vi "App - analyze RUS V6.vi"() -> ()   [LabVIEW 2018] (continued)
"4corners"={"z (-pi/2)"=0.15435451062845643-0.4678200604991372i, "z(inf)"=0.4758200604991372+0.1223545106284564i, "z (pi/2)"=-0.11435451062845639+0.4438200604991372i, "z center"=0.020000000000000018-0.01200000000000001i, "z(0)"=-0.4358200604991372-0.14635451062845642i, "radius"=0.47520844066540857}}, "timestamp(min)"=87.08333333581686, "timestamp"=timestamp(3493733046 s since 1904-01-01), "Magn Field(T)"=0.0}, {"temperature"=210.861, "lorentzian"={"A (VHz)"=0.00034396524768400054, "f (Hz)"=664.2981443004336, "G (Hz)"=0.1690212753358618, "phi(rad)"=-1.2881319002414702, "Q"=3930.2634711541978, "Norm  Ampl"=0.08263262968234714, "bg (V)"=0.48948770996611757+0.12435861413405644i, "4corners"={"z (-pi/2)"=0.15635861413405647-0.48148770996611756i, "z(inf)"=0.48948770996611757+0.12435861413405644i, "z (pi/2)"=-0.11635861413405643+0.45748770996611754i, "z center"=0.020000000000000018-0.01200000000000001i, "z(0)"=-0.44948770996611753-0.14835861413405646i, "radius"=0.488888925480819}}, "timestamp(min)"=88.41666666418314, "timestamp"=timestamp(3493733126 s since 1904-01-01), "Magn Field(T)"=0.0}, {"temperature"=210.594, "lorentzian"={"A (VHz)"=0.0003323733612583622, "f (Hz)"=664.3188476258067, "G (Hz)"=0.16344657299552573, "phi(rad)"=-1.2279818487580703, "Q"=4064.4403577919747, "Norm  Ampl"=0.0788865424699876, "bg (V)"=0.48256027530198187+0.1582356056642887i, "4corners"={"z (-pi/2)"=0.19023560566428874-0.45856027530198185i, "z(inf)"=0.48256027530198187+0.1582356056642887i, "z (pi/2)"=-0.1342356056642887+0.45056027530198184i, "z center"=0.028000000000000025-0.0040000000000000036i, "z(0)"=-0.4265602753019818-0.16623560566428872i, "radius"=0.4826442122597888}}, "timestamp(min)"=89.73333333432674, "timestamp"=timestamp(3493733205 s since 1904-01-01), "Magn Field(T)"=0.0}, {"temperature"=210.336, "lorentzian"={"A (VHz)"=0.00033438773859277484, "f (Hz)"=664.3335964907527, "G (Hz)"=0.16118690371722072, "phi(rad)"=-1.2664496122682602, "Q"=4121.510998537639, "Norm  Ampl"=0.07822762004975677, "bg (V)"=0.4990184327589342+0.13343656181766148i, "4corners"={"z (-pi/2)"=0.18143656181766152-0.4750184327589342i, "z(inf)"=0.4990184327589342+0.13343656181766148i, "z (pi/2)"=-0.10943656181766145+0.45101843275893416i, "z center"=0.03600000000000003-0.01200000000000001i, "z(0)"=-0.42701843275893414-0.1574365618176615i, "radius"=0.4853224315729514}}, "timestamp(min)"=91.0666666701436, "timestamp"=timestamp(3493733285 s since 1904-01-01), "Magn Field(T)"=0.0}, {"temperature"=210.064, "lorentzian"={"A (VHz)"=0.0003264846409159807, "f (Hz)"=664.3536063641833, "G (Hz)"=0.1553160001327941, "phi(rad)"=-1.220684561377293, "Q"=4277.431853744402, "Norm  Ampl"=0.07467473957671357, "bg (V)"=0.4956247544092579+0.16091310841247816i, "4corners"={"z (-pi/2)"=0.2089131084124782-0.45562475440925787i, "z(inf)"=0.4956247544092579+0.16091310841247816i, "z (pi/2)"=-0.12091310841247813+0.44762475440925786i, "z center"=0.04400000000000004-0.0040000000000000036i, "z(0)"=-0.40762475440925783-0.16891310841247817i, "radius"=0.48079231703666836}}, "timestamp(min)"=92.38333333283663, "timestamp"=timestamp(3493733364 s since 1904-01-01), "Magn Field(T)"=0.0}, {"temperature"=209.8, "lorentzian"={"A (VHz)"=0.00033137804714622845, "f (Hz)"=664.3711441248129, "G (Hz)"=0.15484911121026917, "phi(rad)"=-1.2383855845330038, "Q"=4290.442088638566, "Norm  Ampl"=0.07481204115039657, "bg (V)"=0.49268141450734+0.16165586720424824i, "4corners"={"z (-pi/2)"=0.19365586720424827-0.45268141450733995i, "z(inf)"=0.49268141450734+0.16165586720424824i, "z (pi/2)"=-0.1216558672042482+0.46068141450733996i, "z center"=0.03600000000000003+0.0040000000000000036i, "z(0)"=-0.4206814145073399-0.15365586720424823i, "radius"=0.4831286441729039}}, "timestamp(min)"=93.70000000298023, "timestamp"=timestamp(3493733443 s since 1904-01-01), "Magn Field(T)"=0.0}, {"temperature"=209.539, "lorentzian"={"A (VHz)"=0.00035137190295300166, "f (Hz)"=664.3886135894766, "G (Hz)"=0.1587677742828772, "phi(rad)"=-1.2908942860300243, "Q"=4184.656594138132, "Norm  Ampl"=0.07809203185267653, "bg (V)"=0.5007211548751844+0.1478828779205012i, "4corners"={"z (-pi/2)"=0.1638828779205012-0.4607211548751844i, "z(inf)"=0.5007211548751844+0.1478828779205012i, "z (pi/2)"=-0.10788287792050116+0.4847211548751844i, "z center"=0.028000000000000025+0.01200000000000001i, "z(0)"=-0.4447211548751844-0.12388287792050118i, "radius"=0.49186323991378533}}, "timestamp(min)"=95.03333333134651, "timestamp"=timestamp(3493733523 s since 1904-01-01), "Magn Field(T)"=0.0}, {"temperature"=209.267, "lorentzian"={"A (VHz)"=0.0003551473471126149, "f (Hz)"=664.4069577109009, "G (Hz)"=0.15724780606018676, "phi(rad)"=-1.2959877034042098, "Q"=4225.222433034127, "Norm  Ampl"=0.07756980531564582, "bg (V)"=0.5027866875931508+0.14586231534066638i, "4corners"={"z (-pi/2)"=0.1618623153406664-0.46278668759315084i, "z(inf)"=0.5027866875931508+0.14586231534066638i, "z (pi/2)"=-0.10586231534066634+0.48678668759315086i, "z center"=0.028000000000000025+0.01200000000000001i, "z(0)"=-0.4467866875931508-0.12186231534066636i, "radius"=0.4932965823762012}}, "timestamp(min)"=96.35000000149012, "timestamp"=timestamp(3493733602 s since 1904-01-01), "Magn Field(T)"=0.0}, {"temperature"=209.008, "lorentzian"={"A (VHz)"=0.00035824718774550096, "f (Hz)"=664.4245585272355, "G (Hz)"=0.1570614171905534, "phi(rad)"=-1.3013567474955483, "Q"=4230.348677684018, "Norm  Ampl"=0.0778321762150261, "bg (V)"=0.5056730676055248+0.14391175019997515i, "4corners"={"z (-pi/2)"=0.15991175019997517-0.4656730676055247i, "z(inf)"=0.5056730676055248+0.14391175019997515i, "z (pi/2)"=-0.10391175019997512+0.4896730676055247i, "z center"=0.028000000000000025+0.01200000000000001i, "z(0)"=-0.44967306760552467-0.11991175019997513i, "radius"=0.4955524890024192}}, "timestamp(min)"=97.68333333730698, "timestamp"=timestamp(3493733682 s since 1904-01-01), "Magn Field(T)"=0.0}, {"temperature"=208.737, "lorentzian"={"A (VHz)"=0.0003620389778047644, "f (Hz)"=664.4414683185125, "G (Hz)"=0.1572813330614881, "phi(rad)"=-1.315732030850954, "Q"=4224.5411797136385, "Norm  Ampl"=0.07555321252410724, "bg (V)"=0.49282849367948844+0.10120097940000432i, "4corners"={"z (-pi/2)"=0.14920097940000437-0.48482849367948844i, "z(inf)"=0.49282849367948844+0.10120097940000432i, "z (pi/2)"=-0.09320097940000431+0.4448284936794884i, "z center"=0.028000000000000025-0.020000000000000018i, "z(0)"=-0.4368284936794884-0.14120097940000437i, "radius"=0.48036986369240786}}, "timestamp(min)"=99.0, "timestamp"=timestamp(3493733761 s since 1904-01-01), "Magn Field(T)"=0.0}, {"temperature"=208.465, "lorentzian"={"A (VHz)"=0.00036334054298061894, "f (Hz)"=664.4601452577426, "G (Hz)"=0.1577653201754836, "phi(rad)"=-1.3227956670777963, "Q"=4211.699659460383, "Norm  Ampl"=0.07315531107366603, "bg (V)"=0.4775102835579108+0.08582198624427292i, "4corners"={"z (-pi/2)"=0.14182198624427297-0.4775102835579108i, "z(inf)"=0.4775102835579108+0.08582198624427292i, "z (pi/2)"=-0.08582198624427292+0.42151028355791076i, "z center"=0.028000000000000025-0.028000000000000025i, "z(0)"=-0.42151028355791076-0.14182198624427297i, "radius"=0.4636970342550239}}, "timestamp(min)"=100.3166666701436, "timestamp"=timestamp(3493733840 s since 1904-01-01), "Magn Field(T)"=0.0}, {"temperature"=208.205, "lorentzian"={"A (VHz)"=0.0003655921916337196, "f (Hz)"=664.4796852677678, "G (Hz)"=0.15525145365190737, "phi(rad)"=-1.2967215976941358, "Q"=4280.02230985619, "Norm  Ampl"=0.07716533206824039, "bg (V)"=0.5064832255059715+0.13852553307676524i, "4corners"={"z (-pi/2)"=0.16252553307676526-0.4744832255059715i, "z(inf)"=0.5064832255059715+0.13852553307676524i, "z (pi/2)"=-0.10652553307676521+0.4824832255059715i, "z center"=0.028000000000000025+0.0040000000000000036i, "z(0)"=-0.4504832255059715-0.13052553307676523i, "radius"=0.49703452208089755}}, "timestamp(min)"=101.64999999850988, "timestamp"=timestamp(3493733920 s since 1904-01-01), "Magn Field(T)"=0.0}, {"temperature"=207.933, "lorentzian"={"A (VHz)"=0.0003696196043564403, "f (Hz)"=664.4980076667935, "G (Hz)"=0.1551610073255388, "phi(rad)"=-1.3004917013710942, "Q"=4282.635303292595, "Norm  Ampl"=0.07717961611290688, "bg (V)"=0.5073549264995896+0.13682259753273826i, "4corners"={"z (-pi/2)"=0.16082259753273828-0.4753549264995896i, "z(inf)"=0.5073549264995896+0.13682259753273826i, "z (pi/2)"=-0.10482259753273823+0.4833549264995896i, "z center"=0.028000000000000025+0.0040000000000000036i, "z(0)"=-0.4513549264995896-0.12882259753273825i, "radius"=0.49741631253384794}}, "timestamp(min)"=102.96666666865349, "timestamp"=timestamp(3493733999 s since 1904-01-01), "Magn Field(T)"=0.0}, {"temperature"=207.67, "lorentzian"={"A (VHz)"=0.0003688314220528578, "f (Hz)"=664.5154310442224, "G (Hz)"=0.15247576110630867, "phi(rad)"=-1.3185668128316879, "Q"=4358.170939582397, "Norm  Ampl"=0.07594365786598505, "bg (V)"=0.5103106326617382+0.12830020642125523i, "4corners"={"z (-pi/2)"=0.15230020642125525-0.47831063266173807i, "z(inf)"=0.5103106326617382+0.12830020642125523i, "z (pi/2)"=-0.09630020642125518+0.4863106326617381i, "z center"=0.028000000000000025+0.0040000000000000036i, "z(0)"=-0.45431063266173805-0.1203002064212552i, "radius"=0.4980703642006144}}, "timestamp(min)"=104.28333333134651, "timestamp"=timestamp(3493734078 s since 1904-01-01), "Magn Field(T)"=0.0}, {"temperature"=207.397, "lorentzian"={"A (VHz)"=0.00037157271400023234, "f (Hz)"=664.5338643964093, "G (Hz)"=0.15192949142637535, "phi(rad)"=-1.3189009092108237, "Q"=4373.962277879675, "Norm  Ampl"=0.07614323738836301, "bg (V)"=0.5133586305123503+0.1289128189052309i, "4corners"={"z (-pi/2)"=0.15291281890523092-0.4813586305123502i, "z(inf)"=0.5133586305123503+0.1289128189052309i, "z (pi/2)"=-0.09691281890523087+0.48935863051235023i, "z center"=0.028000000000000025+0.0040000000000000036i, "z(0)"=-0.4573586305123502-0.1209128189052309i, "radius"=0.5011748323087215}}, "timestamp(min)"=105.61666666716337, "timestamp"=timestamp(3493734158 s since 1904-01-01), "Magn Field(T)"=0.0}, {"temperature"=207.121, "lorentzian"={"A (VHz)"=0.00037560722465557504, "f (Hz)"=664.5517885931691, "G (Hz)"=0.15163343901734644, "phi(rad)"=-1.3231000954626153, "Q"=4382.620303936695, "Norm  Ampl"=0.07591961547744219, "bg (V)"=0.5133977788844358+0.12675194644126214i, "4corners"={"z (-pi/2)"=0.15075194644126216-0.4813977788844358i, "z(inf)"=0.5133977788844358+0.12675194644126214i, "z (pi/2)"=-0.09475194644126211+0.4893977788844358i, "z center"=0.028000000000000025+0.0040000000000000036i, "z(0)"=-0.4573977788844358-0.11875194644126214i, "radius"=0.5006785836253256}}, "timestamp(min)"=106.93333333730698, "timestamp"=timestamp(3493734237 s since 1904-01-01), "Magn Field(T)"=0.0}, {"temperature"=206.86, "lorentzian"={"A (VHz)"=0.00037939817093463887, "f (Hz)"=664.5704803534437, "G (Hz)"=0.1507306425391779, "phi(rad)"=-1.3256025377721956, "Q"=4408.9938791358145, "Norm  Ampl"=0.07554516623773996, "bg (V)"=0.514202618763606+0.12566179261706728i, "4corners"={"z (-pi/2)"=0.1496617926170673-0.48220261876360593i, "z(inf)"=0.514202618763606+0.12566179261706728i, "z (pi/2)"=-0.09366179261706727+0.49020261876360594i, "z center"=0.028000000000000025+0.0040000000000000036i, "z(0)"=-0.4582026187636059-0.11766179261706729i, "radius"=0.5011931546573503}}, "timestamp(min)"=108.26666666567326, "timestamp"=timestamp(3493734317 s since 1904-01-01), "Magn Field(T)"=0.0}, {"temperature"=206.586, "lorentzian"={"A (VHz)"=0.0003799233187956319, "f (Hz)"=664.588180324614, "G (Hz)"=0.14905726588662013, "phi(rad)"=-1.3374419748250967, "Q"=4458.609758950835, "Norm  Ampl"=0.07486814015789056, "bg (V)"=0.5166640632352237+0.12014782699526805i, "4corners"={"z (-pi/2)"=0.14414782699526807-0.48466406323522376i, "z(inf)"=0.5166640632352237+0.12014782699526805i, "z (pi/2)"=-0.08814782699526802+0.49266406323522377i, "z center"=0.028000000000000025+0.0040000000000000036i, "z(0)"=-0.46066406323522374-0.11214782699526804i, "radius"=0.5022776965118813}}, "timestamp(min)"=109.58333333581686, "timestamp"=timestamp(3493734396 s since 1904-01-01), "Magn Field(T)"=0.0}, {"temperature"=206.322, "lorentzian"={"A (VHz)"=0.00038342258394746456, "f (Hz)"=664.6064246538435, "G (Hz)"=0.14844526330238045, "phi(rad)"=-1.342088405083977, "Q"=4477.114391316425, "Norm  Ampl"=0.0747010798065654, "bg (V)"=0.5181192065643716+0.11809037028339893i, "4corners"={"z (-pi/2)"=0.14209037028339894-0.4861192065643716i, "z(inf)"=0.5181192065643716+0.11809037028339893i, "z (pi/2)"=-0.0860903702833989+0.4941192065643716i, "z center"=0.028000000000000025+0.0040000000000000036i, "z(0)"=-0.46211920656437155-0.11009037028339892i, "radius"=0.5032230611117621}}, "timestamp(min)"=110.89999999850988, "timestamp"=timestamp(3493734475 s since 1904-01-01), "Magn Field(T)"=0.0}, {"temperature"=206.047, "lorentzian"={"A (VHz)"=0.00038522781206593883, "f (Hz)"=664.6239877084581, "G (Hz)"=0.1476327330726419, "phi(rad)"=-1.3521683622314384, "Q"=4501.874170286026, "Norm  Ampl"=0.0739234746791219, "bg (V)"=0.5168062088247101+0.11260258100289335i, "4corners"={"z (-pi/2)"=0.13660258100289335-0.48480620882471004i, "z(inf)"=0.5168062088247101+0.11260258100289335i, "z (pi/2)"=-0.08060258100289332+0.49280620882471005i, "z center"=0.028000000000000025+0.0040000000000000036i, "z(0)"=-0.46080620882471-0.10460258100289334i, "radius"=0.5007255040299785}}, "timestamp(min)"=112.23333333432674, "timestamp"=timestamp(3493734555 s since 1904-01-01), "Magn Field(T)"=0.0}, {"temperature"=205.772, "lorentzian"={"A (VHz)"=0.00038879314280680584, "f (Hz)"=664.6422601490035, "G (Hz)"=0.14766020358391277, "phi(rad)"=-1.3505384031514258, "Q"=4501.160394048208, "Norm  Ampl"=0.07402344475594164, "bg (V)"=0.5171983096693449+0.1135267359741549i, "4corners"={"z (-pi/2)"=0.13752673597415493-0.4851983096693449i, "z(inf)"=0.5171983096693449+0.1135267359741549i, "z (pi/2)"=-0.08152673597415487+0.4931983096693449i, "z center"=0.028000000000000025+0.0040000000000000036i, "z(0)"=-0.4611983096693449-0.10552673597415489i, "radius"=0.5013093776067794}}, "timestamp(min)"=113.55000000447035, "timestamp"=timestamp(3493734634 s since 1904-01-01), "Magn Field(T)"=0.0}, {"temperature"=205.505, "lorentzian"={"A (VHz)"=0.0003927838145535556, "f (Hz)"=664.6602601074228, "G (Hz)"=0.14759958362580006, "phi(rad)"=-1.3539126044269483, "Q"=4503.130996578515, "Norm  Ampl"=0.07397858406419787, "bg (V)"=0.5174693417428737+0.1118543640956627i, "4corners"={"z (-pi/2)"=0.1358543640956627-0.4854693417428737i, "z(inf)"=0.5174693417428737+0.1118543640956627i, "z (pi/2)"=-0.07985436409566267+0.4934693417428737i, "z center"=0.028000000000000025+0.0040000000000000036i, "z(0)"=-0.4614693417428737-0.10385436409566269i, "radius"=0.5012113330329651}}, "timestamp(min)"=114.86666666716337, "timestamp"=timestamp(3493734713 s since 1904-01-01), "Magn Field(T)"=0.0}, {"temperature"=205.23, "lorentzian"={"A (VHz)"=0.0003935754582975437, "f (Hz)"=664.6782562264044, "G (Hz)"=0.14661811059554475, "phi(rad)"=-1.3514260691358269, "Q"=4533.39804698453, "Norm  Ampl"=0.07351191973354369, "bg (V)"=0.5173678077971541+0.11310860545837348i, "4corners"={"z (-pi/2)"=0.1371086054583735-0.48536780779715405i, "z(inf)"=0.5173678077971541+0.11310860545837348i, "z (pi/2)"=-0.08110860545837345+0.49336780779715406i, "z center"=0.028000000000000025+0.0040000000000000036i, "z(0)"=-0.46136780779715403-0.10510860545837347i, "radius"=0.5013836246760193}}, "timestamp(min)"=116.20000000298023, "timestamp"=timestamp(3493734793 s since 1904-01-01), "Magn Field(T)"=0.0}, {"temperature"=204.949, "lorentzian"={"A (VHz)"=0.000399394876662407, "f (Hz)"=664.6963935252326, "G (Hz)"=0.1471833400427258, "phi(rad)"=-1.3610534018832139, "Q"=4516.111628750089, "Norm  Ampl"=0.07359368008705944, "bg (V)"=0.5170555937119127+0.10810707626710435i, "4corners"={"z (-pi/2)"=0.13210707626710438-0.48505559371191265i, "z(inf)"=0.5170555937119127+0.10810707626710435i, "z (pi/2)"=-0.07610707626710432+0.49305559371191265i, "z center"=0.028000000000000025+0.0040000000000000036i, "z(0)"=-0.4610555937119126-0.10010707626710434i, "radius"=0.5000136568832856}}, "timestamp(min)"=117.51666666567326, "timestamp"=timestamp(3493734872 s since 1904-01-01), "Magn Field(T)"=0.0}, {"temperature"=204.683, "lorentzian"={"A (VHz)"=0.00040114335381640425, "f (Hz)"=664.7147754224831, "G (Hz)"=0.14607817985894414, "phi(rad)"=-1.365551239445412, "Q"=4550.404283954963, "Norm  Ampl"=0.07296681070376816, "bg (V)"=0.5170211187425304+0.10580271122694i, "4corners"={"z (-pi/2)"=0.12980271122694004-0.48502111874253045i, "z(inf)"=0.5170211187425304+0.10580271122694i, "z (pi/2)"=-0.07380271122693997+0.49302111874253046i, "z center"=0.028000000000000025+0.0040000000000000036i, "z(0)"=-0.46102111874253043-0.09780271122694i, "radius"=0.49950520176405755}}, "timestamp(min)"=118.85000000149012, "timestamp"=timestamp(3493734952 s since 1904-01-01), "Magn Field(T)"=0.0}, {"temperature"=204.406, "lorentzian"={"A (VHz)"=0.00040274044577660173, "f (Hz)"=664.7329875150317, "G (Hz)"=0.14490265208273315, "phi(rad)"=-1.3769529234230262, "Q"=4587.445281094634, "Norm  Ampl"=0.07263284903932259, "bg (V)"=0.5198648231894291+0.10055717894106385i, "4corners"={"z (-pi/2)"=0.12455717894106387-0.48786482318942903i, "z(inf)"=0.5198648231894291+0.10055717894106385i, "z (pi/2)"=-0.06855717894106382+0.49586482318942904i, "z center"=0.028000000000000025+0.0040000000000000036i, "z(0)"=-0.463864823189429-0.09255717894106384i, "radius"=0.5012527237793576}}, "timestamp(min)"=120.16666666418314, "timestamp"=timestamp(3493735031 s since 1904-01-01), "Magn Field(T)"=0.0}, {"temperature"=204.135, "lorentzian"={"A (VHz)"=0.00040519775284044183, "f (Hz)"=664.7514539650158, "G (Hz)"=0.1448843453340604, "phi(rad)"=-1.381100171905023, "Q"=4588.1523806612495, "Norm  Ampl"=0.07179629292785852, "bg (V)"=0.5146528557763046+0.09743967088502194i, "4corners"={"z (-pi/2)"=0.12143967088502196-0.48265285577630457i, "z(inf)"=0.5146528557763046+0.09743967088502194i, "z (pi/2)"=-0.06543967088502191+0.4906528557763046i, "z center"=0.028000000000000025+0.0040000000000000036i, "z(0)"=-0.45865285577630455-0.08943967088502193i, "radius"=0.4955421012692402}}, "timestamp(min)"=121.48333333432674, "timestamp"=timestamp(3493735110 s since 1904-01-01), "Magn Field(T)"=0.0}, {"temperature"=203.855, "lorentzian"={"A (VHz)"=0.0004062762788775803, "f (Hz)"=664.7696405311139, "G (Hz)"=0.14368029243156008, "phi(rad)"=-1.3844923522740462, "Q"=4626.728059088317, "Norm  Ampl"=0.07145105994855205, "bg (V)"=0.5166866369185976+0.09611245256031146i, "4corners"={"z (-pi/2)"=0.12011245256031149-0.4846866369185976i, "z(inf)"=0.5166866369185976+0.09611245256031146i, "z (pi/2)"=-0.06411245256031144+0.4926866369185976i, "z center"=0.028000000000000025+0.0040000000000000036i, "z(0)"=-0.46068663691859757-0.08811245256031146i, "radius"=0.4972919997541534}}, "timestamp(min)"=122.8166666701436, "timestamp"=timestamp(3493735190 s since 1904-01-01), "Magn Field(T)"=0.0}, {"temperature"=203.577, "lorentzian"={"A (VHz)"=0.00041042061972633404, "f (Hz)"=664.7884789608521, "G (Hz)"=0.14315252563159492, "phi(rad)"=-1.3899343511047206, "Q"=4643.917220655225, "Norm  Ampl"=0.07124545314025889, "bg (V)"=0.5175713074346605+0.09352310091382307i, "4corners"={"z (-pi/2)"=0.11752310091382309-0.4855713074346605i, "z(inf)"=0.5175713074346605+0.09352310091382307i, "z (pi/2)"=-0.06152310091382304+0.4935713074346605i, "z center"=0.028000000000000025+0.0040000000000000036i, "z(0)"=-0.46157130743466046-0.08552310091382306i, "radius"=0.4976891104499971}}, "timestamp(min)"=124.13333333283663, "timestamp"=timestamp(3493735269 s since 1904-01-01), "Magn Field(T)"=0.0}, {"temperature"=203.306, "lorentzian"={"A (VHz)"=0.0004138057215428869, "f (Hz)"=664.8081200534322, "G (Hz)"=0.14252198965919805, "phi(rad)"=-1.395115351872236, "Q"=4664.600330399099, "Norm  Ampl"=0.07081420771256887, "bg (V)"=0.5172172618457117+0.09084142818452332i, "4corners"={"z (-pi/2)"=0.11484142818452334-0.4852172618457117i, "z(inf)"=0.5172172618457117+0.09084142818452332i, "z (pi/2)"=-0.05884142818452329+0.4932172618457117i, "z center"=0.028000000000000025+0.0040000000000000036i, "z(0)"=-0.46121726184571166-0.08284142818452331i, "radius"=0.49686513556189804}}, "timestamp(min)"=125.45000000298023, "timestamp"=timestamp(3493735348 s since 1904-01-01), "Magn Field(T)"=0.0}, {"temperature"=203.002, "lorentzian"={"A (VHz)"=0.0004154653185366444, "f (Hz)"=664.8281506310057, "G (Hz)"=0.1418255973822156, "phi(rad)"=-1.4054415969345646, "Q"=4687.645692330943, "Norm  Ampl"=0.0700233334751772, "bg (V)"=0.5149940155205213+0.08526880650221168i, "4corners"={"z (-pi/2)"=0.1092688065022117-0.4829940155205213i, "z(inf)"=0.5149940155205213+0.08526880650221168i, "z (pi/2)"=-0.05326880650221165+0.4909940155205213i, "z center"=0.028000000000000025+0.0040000000000000036i, "z(0)"=-0.45899401552052127-0.07726880650221167i, "radius"=0.49372845782180275}}, "timestamp(min)"=126.88333333283663, "timestamp"=timestamp(3493735434 s since 1904-01-01), "Magn Field(T)"=0.0}, {"temperature"=202.734, "lorentzian"={"A (VHz)"=0.00041896455878245636, "f (Hz)"=664.8464656256355, "G (Hz)"=0.1411876435021714, "phi(rad)"=-1.4112873255598153, "Q"=4708.956457761195, "Norm  Ampl"=0.07005105188084194, "bg (V)"=0.517857181128416+0.08280612406703723i, "4corners"={"z (-pi/2)"=0.10680612406703725-0.485857181128416i, "z(inf)"=0.517857181128416+0.08280612406703723i, "z (pi/2)"=-0.0508061240670372+0.49385718112841603i, "z center"=0.028000000000000025+0.0040000000000000036i, "z(0)"=-0.461857181128416-0.07480612406703722i, "radius"=0.4961556843305809}}, "timestamp(min)"=128.20000000298023, "timestamp"=timestamp(3493735513 s since 1904-01-01), "Magn Field(T)"=0.0}, {"temperature"=202.449, "lorentzian"={"A (VHz)"=0.0004201254351843168, "f (Hz)"=664.8647360420077, "G (Hz)"=0.14012834414192302, "phi(rad)"=-1.4222845993870865, "Q"=4744.684168740536, "Norm  Ampl"=0.06914144932800301, "bg (V)"=0.5159838369894613+0.07700886817984766i, "4corners"={"z (-pi/2)"=0.10100886817984768-0.48398383698946124i, "z(inf)"=0.5159838369894613+0.07700886817984766i, "z (pi/2)"=-0.04500886817984763+0.49198383698946124i, "z center"=0.028000000000000025+0.0040000000000000036i, "z(0)"=-0.4599838369894612-0.06900886817984765i, "radius"=0.49341515987640616}}, "timestamp(min)"=129.51666666567326, "timestamp"=timestamp(3493735592 s since 1904-01-01), "Magn Field(T)"=0.0}, {"temperature"=202.176, "lorentzian"={"A (VHz)"=0.0004207740570173915, "f (Hz)"=664.8826826665108, "G (Hz)"=0.13778131402834934, "phi(rad)"=-1.4474446636105571, "Q"=4825.637550021531, "Norm  Ampl"=0.06759330264944674, "bg (V)"=0.5148564173047995+0.06436100342319324i, "4corners"={"z (-pi/2)"=0.08836100342319327-0.48285641730479945i, "z(inf)"=0.5148564173047995+0.06436100342319324i, "z (pi/2)"=-0.032361003423193216+0.49085641730479945i, "z center"=0.028000000000000025+0.0040000000000000036i, "z(0)"=-0.4588564173047994-0.05636100342319324i, "radius"=0.4905839599957583}}, "timestamp(min)"=130.85000000149012, "timestamp"=timestamp(3493735672 s since 1904-01-01), "Magn Field(T)"=0.0}, {"temperature"=201.892, "lorentzian"={"A (VHz)"=0.00042618732161807523, "f (Hz)"=664.9021630370361, "G (Hz)"=0.13795986030766882, "phi(rad)"=-1.4333809252013117, "Q"=4819.533461067704, "Norm  Ampl"=0.06811496040998716, "bg (V)"=0.5170760577643687+0.07163282312271847i, "4corners"={"z (-pi/2)"=0.0956328231227185-0.4850760577643687i, "z(inf)"=0.5170760577643687+0.07163282312271847i, "z (pi/2)"=-0.039632823122718444+0.4930760577643687i, "z center"=0.028000000000000025+0.0040000000000000036i, "z(0)"=-0.46107605776436866-0.06363282312271847i, "radius"=0.4937302796486002}}, "timestamp(min)"=132.16666666418314, "timestamp"=timestamp(3493735751 s since 1904-01-01), "Magn Field(T)"=0.0}, {"temperature"=201.608, "lorentzian"={"A (VHz)"=0.0004222053109160282, "f (Hz)"=664.9200138534414, "G (Hz)"=0.13455598213025302, "phi(rad)"=-1.4568903173145586, "Q"=4941.586418727819, "Norm  Ampl"=0.0656738771838343, "bg (V)"=0.5129155804493046+0.05147492776327568i, "4corners"={"z (-pi/2)"=0.08347492776327571-0.48891558044930467i, "z(inf)"=0.5129155804493046+0.05147492776327568i, "z (pi/2)"=-0.02747492776327566+0.48091558044930466i, "z center"=0.028000000000000025-0.0040000000000000036i, "z(0)"=-0.45691558044930464-0.05947492776327569i, "radius"=0.48807846477060096}}, "timestamp(min)"=133.48333333432674, "timestamp"=timestamp(3493735830 s since 1904-01-01), "Magn Field(T)"=0.0}, {"temperature"=201.335, "lorentzian"={"A (VHz)"=0.00043527155775633297, "f (Hz)"=664.9394190348338, "G (Hz)"=0.13755032667462308, "phi(rad)"=-1.437200578199426, "Q"=4834.15368840058, "Norm  Ampl"=0.06784906485367707, "bg (V)"=0.5168718725621029+0.06970255219795153i, "4corners"={"z (-pi/2)"=0.09370255219795155-0.4848718725621029i, "z(inf)"=0.5168718725621029+0.06970255219795153i, "z (pi/2)"=-0.0377025521979515+0.4928718725621029i, "z center"=0.028000000000000025+0.0040000000000000036i, "z(0)"=-0.4608718725621029-0.061702552197951524i, "radius"=0.4932672025866929}}, "timestamp(min)"=134.8166666701436, "timestamp"=timestamp(3493735910 s since 1904-01-01), "Magn Field(T)"=0.0}, {"temperature"=201.049, "lorentzian"={"A (VHz)"=0.0004337329085345937, "f (Hz)"=664.9570161356205, "G (Hz)"=0.13599300285722027, "phi(rad)"=-1.4572140613302493, "Q"=4889.641394519115, "Norm  Ampl"=0.06707327717847487, "bg (V)"=0.5180332138674804+0.059899675538049535i, "4corners"={"z (-pi/2)"=0.08389967553804956-0.4860332138674804i, "z(inf)"=0.5180332138674804+0.059899675538049535i, "z (pi/2)"=-0.027899675538049507+0.4940332138674804i, "z center"=0.028000000000000025+0.0040000000000000036i, "z(0)"=-0.46203321386748036-0.05189967553804953i, "radius"=0.4932112371170703}}, "timestamp(min)"=136.13333333283663, "timestamp"=timestamp(3493735989 s since 1904-01-01), "Magn Field(T)"=0.0}, {"temperature"=200.772, "lorentzian"={"A (VHz)"=0.00043536736981719925, "f (Hz)"=664.9751037863994, "G (Hz)"=0.1353871804852172, "phi(rad)"=-1.4711877739865447, "Q"=4911.65486572052, "Norm  Ampl"=0.0664737474009468, "bg (V)"=0.5165562133911143+0.05282596582311021i, "4corners"={"z (-pi/2)"=0.07682596582311023-0.4845562133911143i, "z(inf)"=0.5165562133911143+0.05282596582311021i, "z (pi/2)"=-0.02082596582311018+0.49255621339111433i, "z center"=0.028000000000000025+0.0040000000000000036i, "z(0)"=-0.4605562133911143-0.0448259658231102i, "radius"=0.4909899679032388}}, "timestamp(min)"=137.4666666686535, "timestamp"=timestamp(3493736069 s since 1904-01-01), "Magn Field(T)"=0.0}, {"temperature"=200.485, "lorentzian"={"A (VHz)"=0.0004393784355718948, "f (Hz)"=664.9946492766225, "G (Hz)"=0.13605215179476612, "phi(rad)"=-1.460181607044695, "Q"=4887.792221616332, "Norm  Ampl"=0.06650378434323737, "bg (V)"=0.5138235666004954+0.04995949327843271i, "4corners"={"z (-pi/2)"=0.08195949327843274-0.4898235666004954i, "z(inf)"=0.5138235666004954+0.04995949327843271i, "z (pi/2)"=-0.025959493278432687+0.4818235666004954i, "z center"=0.028000000000000025-0.0040000000000000036i, "z(0)"=-0.4578235666004954-0.057959493278432715i, "radius"=0.4888109703958078}}, "timestamp(min)"=138.7833333313465, "timestamp"=timestamp(3493736148 s since 1904-01-01), "Magn Field(T)"=0.0}, {"temperature"=200.196, "lorentzian"={"A (VHz)"=0.0004439993589116813, "f (Hz)"=665.013363493181, "G (Hz)"=0.13613525265981952, "phi(rad)"=-1.467072549665521, "Q"=4884.94604079477, "Norm  Ampl"=0.06617207297215337, "bg (V)"=0.511463544896849+0.04632727861916547i, "4corners"={"z (-pi/2)"=0.0783272786191655-0.487463544896849i, "z(inf)"=0.511463544896849+0.04632727861916547i, "z (pi/2)"=-0.022327278619165447+0.479463544896849i, "z center"=0.028000000000000025-0.0040000000000000036i, "z(0)"=-0.455463544896849-0.054327278619165476i, "radius"=0.4860759551936699}}, "timestamp(min)"=140.10000000149012, "timestamp"=timestamp(3493736227 s since 1904-01-01), "Magn Field(T)"=0.0}, {"temperature"=199.92, "lorentzian"={"A (VHz)"=0.00044238402185645966, "f (Hz)"=665.0319666327775, "G (Hz)"=0.13289238047804208, "phi(rad)"=-1.4762596135382466, "Q"=5004.289668380658, "Norm  Ampl"=0.06523251554991082, "bg (V)"=0.5166753826768884+0.04233588437882818i, "4corners"={"z (-pi/2)"=0.07433588437882821-0.4926753826768884i, "z(inf)"=0.5166753826768884+0.04233588437882818i, "z (pi/2)"=-0.01833588437882816+0.48467538267688837i, "z center"=0.028000000000000025-0.0040000000000000036i, "z(0)"=-0.46067538267688835-0.05033588437882819i, "radius"=0.49086723644542773}}, "timestamp(min)"=141.43333333730698, "timestamp"=timestamp(3493736307 s since 1904-01-01), "Magn Field(T)"=0.0}, {"temperature"=199.633, "lorentzian"={"A (VHz)"=0.00044487810801382684, "f (Hz)"=665.0514303799941, "G (Hz)"=0.13201590294735027, "phi(rad)"=-1.478215534764768, "Q"=5037.661490261712, "Norm  Ampl"=0.06469246807790581, "bg (V)"=0.5159368202695078+0.04130308528292976i, "4corners"={"z (-pi/2)"=0.07330308528292978-0.4919368202695078i, "z(inf)"=0.5159368202695078+0.04130308528292976i, "z (pi/2)"=-0.017303085282929738+0.4839368202695078i, "z center"=0.028000000000000025-0.0040000000000000036i, "z(0)"=-0.4599368202695078-0.049303085282929766i, "radius"=0.4900354172005023}}, "timestamp(min)"=142.75, "timestamp"=timestamp(3493736386 s since 1904-01-01), "Magn Field(T)"=0.0}, {"temperature"=199.352, "lorentzian"={"A (VHz)"=0.00044791112692119095, "f (Hz)"=665.070428839104, "G (Hz)"=0.13144453878155832, "phi(rad)"=-1.4924649400075496, "Q"=5059.7037731963455, "Norm  Ampl"=0.0640936695377525, "bg (V)"=0.5141148092218479+0.0341561186010366i, "4corners"={"z (-pi/2)"=0.06615611860103662-0.49011480922184797i, "z(inf)"=0.5141148092218479+0.0341561186010366i, "z (pi/2)"=-0.01015611860103658+0.48211480922184796i, "z center"=0.028000000000000025-0.0040000000000000036i, "z(0)"=-0.45811480922184794-0.04215611860103661i, "radius"=0.48760998465114513}}, "timestamp(min)"=144.0666666701436, "timestamp"=timestamp(3493736465 s since 1904-01-01), "Magn Field(T)"=0.0}, {"temperature"=199.061, "lorentzian"={"A (VHz)"=0.00045047575077157364, "f (Hz)"=665.0899681894765, "G (Hz)"=0.130795364655206, "phi(rad)"=-1.4968074971462784, "Q"=5084.96589265791, "Norm  Ampl"=0.06376749766742552, "bg (V)"=0.5142025098836627+0.032039342646732145i, "4corners"={"z (-pi/2)"=0.06403934264673217-0.49020250988366265i, "z(inf)"=0.5142025098836627+0.032039342646732145i, "z (pi/2)"=-0.008039342646732124+0.48220250988366264i, "z center"=0.028000000000000025-0.0040000000000000036i, "z(0)"=-0.4582025098836626-0.04003934264673215i, "radius"=0.4875363728334345}}, "timestamp(min)"=145.39999999850988, "timestamp"=timestamp(3493736545 s since 1904-01-01), "Magn Field(T)"=0.0}, {"temperature"=198.769, "lorentzian"={"A (VHz)"=0.00045177203449588697, "f (Hz)"=665.1092165846538, "G (Hz)"=0.13001905546291714, "phi(rad)"=-1.500739091448192, "Q"=5115.4749141701795, "Norm  Ampl"=0.06340742298006159, "bg (V)"=0.5144816472912067+0.030137426552997178i, "4corners"={"z (-pi/2)"=0.062137426552997206-0.4904816472912067i, "z(inf)"=0.5144816472912067+0.030137426552997178i, "z (pi/2)"=-0.006137426552997156+0.4824816472912067i, "z center"=0.028000000000000025-0.0040000000000000036i, "z(0)"=-0.45848164729120666-0.038137426552997185i, "radius"=0.4876779234728873}}, "timestamp(min)"=146.7166666686535, "timestamp"=timestamp(3493736624 s since 1904-01-01), "Magn Field(T)"=0.0}, {"temperature"=198.49, "lorentzian"={"A (VHz)"=0.0004563703364526659, "f (Hz)"=665.128636002681, "G (Hz)"=0.13008286714925255, "phi(rad)"=-1.5005780440832663, "Q"=5113.114821181913, "Norm  Ampl"=0.0632670226082271, "bg (V)"=0.51316084898709+0.030123262900490708i, "4corners"={"z (-pi/2)"=0.062123262900490736-0.48916084898709i, "z(inf)"=0.51316084898709+0.030123262900490708i, "z (pi/2)"=-0.006123262900490686+0.48116084898709i, "z center"=0.028000000000000025-0.0040000000000000036i, "z(0)"=-0.45716084898709-0.038123262900490715i, "radius"=0.4863593799453753}}, "timestamp(min)"=148.05000000447035, "timestamp"=timestamp(3493736704 s since 1904-01-01), "Magn Field(T)"=0.0}, {"temperature"=198.198, "lorentzian"={"A (VHz)"=0.00045847001179977355, "f (Hz)"=665.1480453032892, "G (Hz)"=0.12876072637020372, "phi(rad)"=-1.5124261491685282, "Q"=5165.768041653499, "Norm  Ampl"=0.06286923339753725, "bg (V)"=0.5154325067280124+0.024483878276874975i, "4corners"={"z (-pi/2)"=0.056483878276875-0.4914325067280124i, "z(inf)"=0.5154325067280124+0.024483878276874975i, "z (pi/2)"=-0.0004838782768749536+0.4834325067280124i, "z center"=0.028000000000000025-0.0040000000000000036i, "z(0)"=-0.4594325067280124-0.03248387827687498i, "radius"=0.48826404735229656}}, "timestamp(min)"=149.36666666716337, "timestamp"=timestamp(3493736783 s since 1904-01-01), "Magn Field(T)"=0.0}, {"temperature"=197.916, "lorentzian"={"A (VHz)"=0.00045832995290242883, "f (Hz)"=665.1669866582076, "G (Hz)"=0.1277616436721843, "phi(rad)"=-1.528843939192106, "Q"=5206.312063148769, "Norm  Ampl"=0.061880747051761054, "bg (V)"=0.511919102135742+0.016313480400689095i, "4corners"={"z (-pi/2)"=0.04831348040068913-0.48791910213574197i, "z(inf)"=0.511919102135742+0.016313480400689095i, "z (pi/2)"=0.007686519599310927+0.47991910213574196i, "z center"=0.028000000000000025-0.0040000000000000036i, "z(0)"=-0.45591910213574194-0.024313480400689102i, "radius"=0.48434526414310264}}, "timestamp(min)"=150.68333333730698, "timestamp"=timestamp(3493736862 s since 1904-01-01), "Magn Field(T)"=0.0}, {"temperature"=197.62, "lorentzian"={"A (VHz)"=0.0004615739940061162, "f (Hz)"=665.185992115189, "G (Hz)"=0.12913793169670015, "phi(rad)"=-1.5312291689362665, "Q"=5150.972943236216, "Norm  Ampl"=0.06233580514581389, "bg (V)"=0.5103293626600669+0.015094367531599057i, "4corners"={"z (-pi/2)"=0.04709436753159908-0.4863293626600668i, "z(inf)"=0.5103293626600669+0.015094367531599057i, "z (pi/2)"=0.008905632468400964+0.4783293626600668i, "z center"=0.028000000000000025-0.0040000000000000036i, "z(0)"=-0.4543293626600668-0.023094367531599064i, "radius"=0.48270716687811677}}, "timestamp(min)"=152.01666666567326, "timestamp"=timestamp(3493736942 s since 1904-01-01), "Magn Field(T)"=0.0}, {"temperature"=197.325, "lorentzian"={"A (VHz)"=0.0004599859942757351, "f (Hz)"=665.2049981978538, "G (Hz)"=0.127257388454758, "phi(rad)"=-1.5546331169239278, "Q"=5227.240683430688, "Norm  Ampl"=0.06140538376567874, "bg (V)"=0.5104659976715589+0.003798878338441551i, "4corners"={"z (-pi/2)"=0.03579887833844158-0.48646599767155885i, "z(inf)"=0.5104659976715589+0.003798878338441551i, "z (pi/2)"=0.02020112166155847+0.47846599767155884i, "z center"=0.028000000000000025-0.0040000000000000036i, "z(0)"=-0.4544659976715588-0.011798878338441558i, "radius"=0.48252902649742263}}, "timestamp(min)"=153.33333333581686, "timestamp"=timestamp(3493737021 s since 1904-01-01), "Magn Field(T)"=0.0}, {"temperature"=197.042, "lorentzian"={"A (VHz)"=0.0004652071057005847, "f (Hz)"=665.2252219651873, "G (Hz)"=0.12756701635047923, "phi(rad)"=-1.5413065620691433, "Q"=5214.711772653984, "Norm  Ampl"=0.061806965550151347, "bg (V)"=0.5122951898390481+0.010285892670484617i, "4corners"={"z (-pi/2)"=0.042285892670484646-0.48829518983904807i, "z(inf)"=0.5122951898390481+0.010285892670484617i, "z (pi/2)"=0.013714107329515404+0.48029518983904806i, "z center"=0.028000000000000025-0.0040000000000000036i, "z(0)"=-0.45629518983904804-0.018285892670484624i, "radius"=0.48450584891271664}}, "timestamp(min)"=154.64999999850988, "timestamp"=timestamp(3493737100 s since 1904-01-01), "Magn Field(T)"=0.0}, {"temperature"=196.746, "lorentzian"={"A (VHz)"=0.0004673461309212847, "f (Hz)"=665.2450117111404, "G (Hz)"=0.12755349714072203, "phi(rad)"=-1.5457693577856824, "Q"=5215.419620970611, "Norm  Ampl"=0.061328025281346024, "bg (V)"=0.5086518149563024+0.008031770211827343i, "4corners"={"z (-pi/2)"=0.04003177021182737-0.48465181495630233i, "z(inf)"=0.5086518149563024+0.008031770211827343i, "z (pi/2)"=0.01596822978817268+0.4766518149563023i, "z center"=0.028000000000000025-0.0040000000000000036i, "z(0)"=-0.4526518149563023-0.016031770211827348i, "radius"=0.4808023821854647}}, "timestamp(min)"=155.98333333432674, "timestamp"=timestamp(3493737180 s since 1904-01-01), "Magn Field(T)"=0.0}, {"temperature"=196.459, "lorentzian"={"A (VHz)"=0.0004653341111726216, "f (Hz)"=665.2636719185228, "G (Hz)"=0.12544868567168027, "phi(rad)"=-1.5698197617134113, "Q"=5303.074068544861, "Norm  Ampl"=0.06041362198027647, "bg (V)"=0.5095801205823622-0.0035297055207983413i, "4corners"={"z (-pi/2)"=0.028470294479201685-0.48558012058236216i, "z(inf)"=0.5095801205823622-0.0035297055207983413i, "z (pi/2)"=0.027529705520798364+0.47758012058236216i, "z center"=0.028000000000000025-0.0040000000000000036i, "z(0)"=-0.45358012058236213-0.004470294479201666i, "radius"=0.48158035021896356}}, "timestamp(min)"=157.30000000447035, "timestamp"=timestamp(3493737259 s since 1904-01-01), "Magn Field(T)"=0.0}, {"temperature"=196.161, "lorentzian"={"A (VHz)"=0.0004668535432705484, "f (Hz)"=665.2820790020305, "G (Hz)"=0.12485198988822187, "phi(rad)"=4.705832603292771, "Q"=5328.566085311477, "Norm  Ampl"=0.06024791729427062, "bg (V)"=0.5105443506501866-0.007163788059516892i, "4corners"={"z (-pi/2)"=0.024836211940483136-0.48654435065018653i, "z(inf)"=0.5105443506501866-0.007163788059516892i, "z (pi/2)"=0.031163788059516914+0.4785443506501865i, "z center"=0.028000000000000025-0.0040000000000000036i, "z(0)"=-0.4545443506501865-0.0008362119404831145i, "radius"=0.4825547221811178}}, "timestamp(min)"=158.63333333283663, "timestamp"=timestamp(3493737339 s since 1904-01-01), "Magn Field(T)"=0.0}, {"temperature"=195.862, "lorentzian"={"A (VHz)"=0.0004698190137035185, "f (Hz)"=665.302621721353, "G (Hz)"=0.12481633057219292, "phi(rad)"=4.708694878956189, "Q"=5330.2530099340365, "Norm  Ampl"=0.059815011929151216, "bg (V)"=0.5072209763422528-0.005770298946008025i, "4corners"={"z (-pi/2)"=0.026229701053992003-0.48322097634225286i, "z(inf)"=0.5072209763422528-0.005770298946008025i, "z (pi/2)"=0.029770298946008047+0.47522097634225285i, "z center"=0.028000000000000025-0.0040000000000000036i, "z(0)"=-0.45122097634225283-0.0022297010539919825i, "radius"=0.479224246177904}}, "timestamp(min)"=159.95000000298023, "timestamp"=timestamp(3493737418 s since 1904-01-01), "Magn Field(T)"=0.0}, {"temperature"=195.573, "lorentzian"={"A (VHz)"=0.0004695194217306301, "f (Hz)"=665.3209060628186, "G (Hz)"=0.12361101586862246, "phi(rad)"=4.686315969271938, "Q"=5382.375522016111, "Norm  Ampl"=0.05913198313777316, "bg (V)"=0.5062088784197923-0.016471171504734344i, "4corners"={"z (-pi/2)"=0.015528828495265684-0.4822088784197923i, "z(inf)"=0.5062088784197923-0.016471171504734344i, "z (pi/2)"=0.040471171504734366+0.4742088784197923i, "z center"=0.028000000000000025-0.0040000000000000036i, "z(0)"=-0.4502088784197923+0.008471171504734337i, "radius"=0.4783714681272455}}, "timestamp(min)"=161.26666666567326, "timestamp"=timestamp(3493737497 s since 1904-01-01), "Magn Field(T)"=0.0}, {"temperature"=195.277, "lorentzian"={"A (VHz)"=0.00046961329043416757, "f (Hz)"=665.3411726525135, "G (Hz)"=0.123149899681447, "phi(rad)"=4.679716724347356, "Q"=5402.693582159285, "Norm  Ampl"=0.05877340427319146, "bg (V)"=0.5049962266073525-0.019590090590190602i, "4corners"={"z (-pi/2)"=0.012409909409809424-0.48099622660735253i, "z(inf)"=0.5049962266073525-0.019590090590190602i, "z (pi/2)"=0.043590090590190624+0.4729962266073525i, "z center"=0.028000000000000025-0.0040000000000000036i, "z(0)"=-0.4489962266073525+0.011590090590190597i, "radius"=0.47725093098103344}}, "timestamp(min)"=162.60000000149012, "timestamp"=timestamp(3493737577 s since 1904-01-01), "Magn Field(T)"=0.0}, {"temperature"=194.992, "lorentzian"={"A (VHz)"=0.00047544919830813415, "f (Hz)"=665.3602455630045, "G (Hz)"=0.1236194283901668, "phi(rad)"=4.6758528074998, "Q"=5382.327472531251, "Norm  Ampl"=0.05913141926985548, "bg (V)"=0.5060151259584926-0.021472618661467754i, "4corners"={"z (-pi/2)"=0.010527381338532274-0.48201512595849266i, "z(inf)"=0.5060151259584926-0.021472618661467754i, "z (pi/2)"=0.045472618661467776+0.47401512595849266i, "z center"=0.028000000000000025-0.0040000000000000036i, "z(0)"=-0.45001512595849263+0.013472618661467747i, 
